vi "Hexapod-connect.vi"(0 "IP":string, 7 "Port":u16, 11 "Signature":u32=9518, 13 "path_config":path=path "C:/BonOMM/BonOMM 7.1/BonOMM 7.1.vi") -> (4 "connection ID":refnum<k5>, 6 "Connexion":bool, 8 "Lecture":bool, 10 "Écriture":bool, 15 "Error OUT":errorcluster)   [LabVIEW 2011]
panel:
  out "SignatureReturned":u32
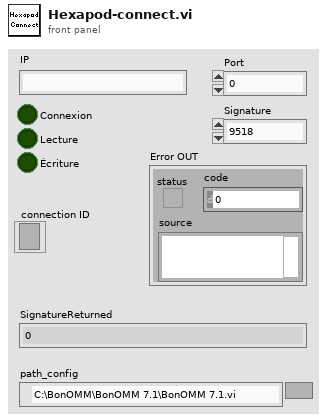
[diagram p1: front panel]
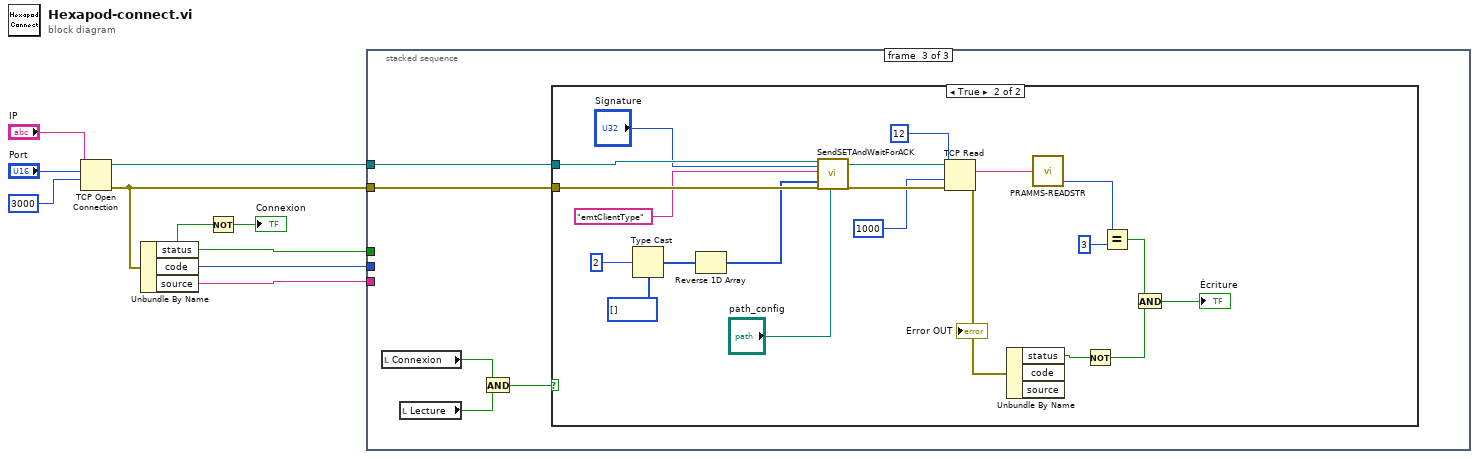
[diagram p0: block diagram]
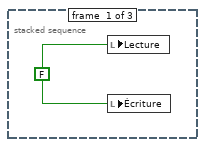
[diagram p2: hidden frame]
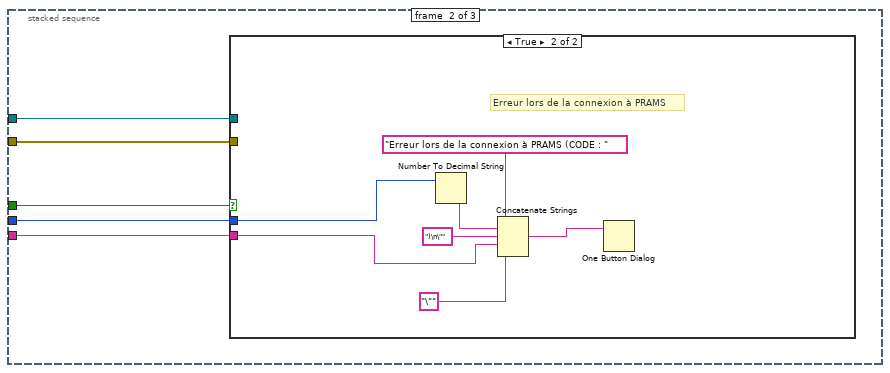
[diagram p3: hidden frame]
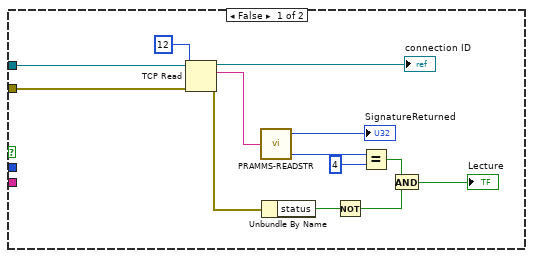
[diagram p4: hidden frame]
diagram:
  n1 = TCP Open Connection(address="IP", remote port or service name="Port", timeout ms (60000)=3000) -> (connection ID=w9:refnum<k5>, error out=w6:errorcluster)  [unwired: 2 in]
  n2 = Unbundle By Name(w6) -> ("status"=w2:bool, "code"=w5:i32, "source"=w4:string)
  n3 = Not(x=w2) -> (.not. x?=→"Connexion":bool)
  n4 = stacked-sequence {
    tunnel: w9 -> [_ w15 w36]
    tunnel: w6 -> [_ w14 w37]
    tunnel: w5 -> [_ w13 _]
    tunnel: w4 -> [_ w12 _]
    tunnel: w2 -> [_ w11 _]
    frame #0 {
      w10 = FALSE
      n5 = local write "Lecture"(w10) -> ()
      n6 = local write "Écriture"(w10) -> ()
    }
    frame #1 {
      n7 = case shown="True" w11 {
        tunnel: w15 -> [w27 _]
        tunnel: w14 -> [w26 _]
        tunnel: w13 -> [_ w35]
        tunnel: w12 -> [_ w30]
        frame False {
          n8 = TCP Read(connection ID=w27, bytes to read=12, error in (no error)=w26) -> (connection ID out=→"connection ID":refnum<k5>, data out=w25:string, error out=w18:errorcluster)  [unwired: 2 in]
          n9 = call "PRAMMS-READSTR.vi"("String"=w25) -> ("Signature"=→"SignatureReturned":u32, "Type"=w24:u32)  [unwired: 1 out]
          n10 = Unbundle By Name(w18) -> ("status"=w22:bool)
          n11 = Not(x=w22) -> (.not. x?=w21:bool)
          n12 = Equal?(x=w24, y=u32 4) -> (x = y?=w20:bool)
          n13 = And(x=w20, y=w21) -> (x .and. y?=→"Lecture":bool)
        }
        frame True {
          # "Erreur lors de la connexion à PRAMS"
          n14 = Number To Decimal String(number=w35) -> (decimal integer string=w34:string)  [unwired: 1 in]
          n15 = Concatenate Strings("Erreur lors de la connexion à PRAMS (CODE : ", w34, ")\n\"", w30, "\"") -> (w31:string)
          n16 = One Button Dialog(message=w31) -> ()  [unwired: 1 in, 1 out]
        }
      }
    }
    frame #2 {
      n17 = local read "Connexion"() -> (w40:bool)
      n18 = local read "Lecture"() -> (w39:bool)
      n19 = And(x=w40, y=w39) -> (x .and. y?=w38:bool)
      n20 = case shown="True" w38 {
        tunnel: w37 -> [_ w60]
        tunnel: w36 -> [_ w61]
        frame False {
        }
        frame True {
          n21 = Type Cast(type=u8[] [], x=u32 2) -> (*(type *) &x=w56:u8[])
          n22 = Reverse 1D Array(array=w56) -> (reversed array=w55:u8[])
          n23 = call "SendSETAndWaitForACK.vi"("connection ID"=w61, "Signature"="Signature", "Active SET"="emtClientType", "Value (little endianed byte array)"=w55, "Error IN"=w60, "path_config"="path_config") -> ("connection ID (dup)"=w50:refnum<k5>, "Error OUT"=w49:errorcluster)  [unwired: 12 in]
          n24 = TCP Read(connection ID=w50, bytes to read=12, error in (no error)=w49, 9:1000 ("timeout ms (25000)")) -> (data out=w51:string, error out=w48:errorcluster)  [unwired: 1 in, 1 out]
          "Error OUT" <- w48
          n25 = Unbundle By Name(w48) -> ("status"=w53:bool)  [unwired: 2 out]
          n26 = call "PRAMMS-READSTR.vi"("String"=w51) -> ("Type"=w47:u32)  [unwired: 2 out]
          n27 = Not(x=w53) -> (.not. x?=w44:bool)
          n28 = Equal?(x=w47, y=u32 3) -> (x = y?=w45:bool)
          n29 = And(x=w45, y=w44) -> (x .and. y?=→"Écriture":bool)
        }
      }
    }
  }
